vi "Export File - Tx XML.vi"(6 "RootNode":refnum<k24>, 7 "Tx Packets":T1 {"Tx Packet Data"."Endianness" items=["big-endian"=0, "little-endian"=2]}, 8 "error in (no error)":errorcluster, 11 "XmlDocument in":refnum<k24>) -> (0 "error out":errorcluster, 3 "XmlDocument out":refnum<k24>)   [LabVIEW 2016, in "UDP-Custom-Device System Explorer.lvlib"]
uses:
  UDP-Custom-Device System Explorer.lvlib
  System.Xml
  Types/XML - New/ImpExp - Tx Packets Data.ctl
  <vilib>/NI Veristand/Custom Device API/Custom Device Item Info.ctl
  Types/XML - New/ImpExp - Tx Packet Data.ctl
  Shared/Types/Shared - Channel Data Type.ctl
  Shared/Types/Shared - Buffered.PacketInfo.ctl
  Shared/Types/Shared - Pointer Encoding.ctl
  Types/XML - New/ImpExp - Packet Headers.ctl
  <vilib>/NI VeriStand/Custom Device API/Custom Device API.lvlib
  Shared/UDP-Custom-Device Shared.lvlib
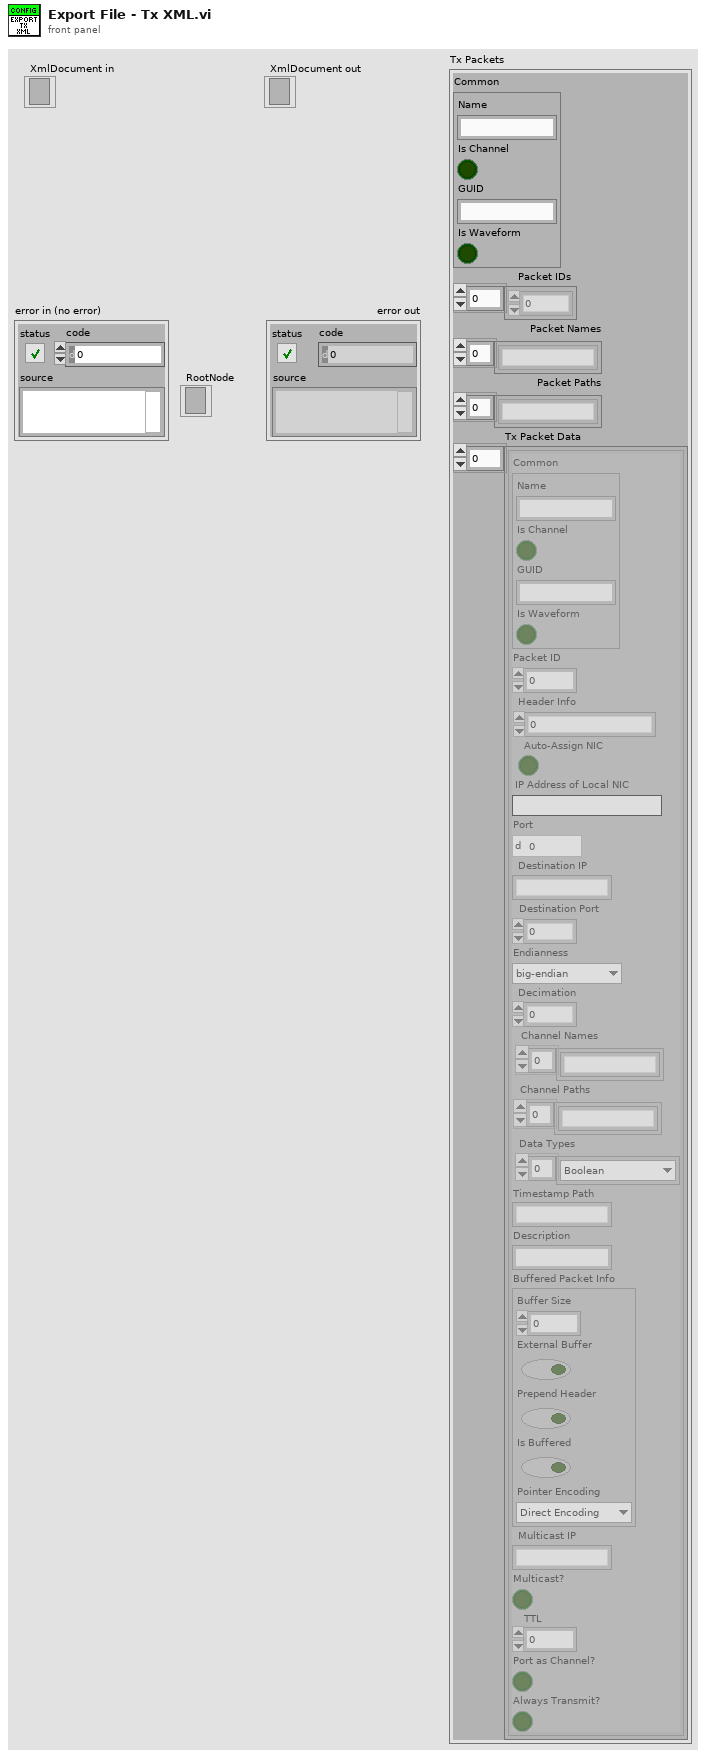
[diagram p1: front panel]
types:
  T1 = typedef "UDP-Custom-Device System Explorer.lvlib/ImpExp - Tx Packets Data.ctl" = cluster{"Common":T2, "Packet IDs":i32[], "Packet Names":string[], "Packet Paths":string[], "Tx Packet Data":T3[]}
  T2 = typedef "Custom Device API.lvlib/Custom Device Item Info.ctl" = cluster{"Name":string, "Is Channel":bool, "GUID":string, "Is Waveform":bool}
  T3 = typedef "UDP-Custom-Device System Explorer.lvlib/ImpExp - Tx Packet Data.ctl" = cluster{"Common":T2, "Packet ID":i32, "Header Info":u32, "Auto-Assign NIC":bool, "IP Address of Local NIC":string, "Port":u16, "Destination IP":string, "Destination Port":u16, "Endianness":u16, "Decimation":u16, "Channel Names":string[], "Channel Paths":string[], "Data Types":T4[], "Timestamp Path":string, "Description":string, "Buffered Packet Info":T5, "Multicast IP":string, "Multicast?":bool, "TTL":u16, "Port as Channel?":bool, "Always Transmit?":bool}
  T4 = typedef "UDP-Custom-Device Shared.lvlib/Shared - Channel Data Type.ctl" = enum16{"Boolean", "Single", "Double", "I8", "I16", "I32", "I64", "U8", "U16", "U32", "U64"}
  T5 = typedef "UDP-Custom-Device Shared.lvlib/Shared - Buffered.PacketInfo.ctl" = cluster{"Buffer Size":i32, "External Buffer":bool, "Prepend Header":bool, "Is Buffered":bool, "Pointer Encoding":T6}
  T6 = typedef "UDP-Custom-Device Shared.lvlib/Shared - Pointer Encoding.ctl" = enum16{"Direct Encoding", "Conversion Encoding"}
  T7 = typedef "UDP-Custom-Device System Explorer.lvlib/ImpExp - Packet Headers.ctl" = cluster{"Packet Name":string, "Packet ID":string, "Packet Path":string}
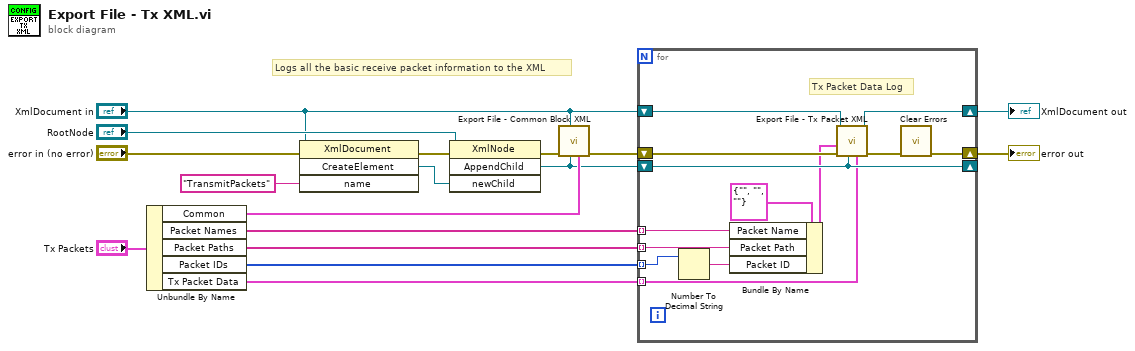
[diagram p0: block diagram]
diagram:
  # "Logs all the basic receive packet information to the XML"
  n1 = Unbundle By Name("Tx Packets") -> ("Common"=w10:T2, "Packet Names"=w6:string[], "Packet Paths"=w5:string[], "Packet IDs"=w4:i32[], "Tx Packet Data"=w3:T3[])
  n2 = invoke class="XmlDocument" method="CreateElement"(reference="XmlDocument in", error in="error in (no error)", "name"="TransmitPackets" ("Tag Name")) -> (error out=w15:errorcluster, "CreateElement"=w16:refnum<k24>)  [unwired: 1 in, 2 out]
  n3 = invoke class="XmlNode" method="AppendChild"(reference="RootNode", error in=w15, "newChild"=w16) -> (error out=w14:errorcluster, "AppendChild"=w7:refnum<k24>)  [unwired: 1 in, 2 out]
  n4 = call "Export File - Common Block XML.vi"("Common"=w10, "RootNode in"=w7, "XmlDocument in"="XmlDocument in", "error in (no error)"=w14) -> ("error out"=w8:errorcluster)  [unwired: 7 in]
  n5 = for {
    shift-right: [w18] -> w1
    shift-left: w8 -> [w25]
    shift-right: [w23] -> w2
    shift-left: "XmlDocument in" -> [w24]
    tunnel: w6 -> [w29] mode=indexing
    tunnel: w4 -> [w28] mode=indexing
    shift-right: [w22] -> _
    shift-left: w7 -> [w22]
    tunnel: w3 -> [w21] mode=indexing
    tunnel: w5 -> [w26] mode=indexing
    # "Tx Packet Data Log"
    n6 = Number To Decimal String(number=w28) -> (decimal integer string=w27:string)  [unwired: 1 in]
    n7 = Bundle By Name(cluster=T7 {"Packet Name"="", "Packet ID"="", "Packet Path"=""} ("Rx Packet XML Data"), "Packet Name"=w29, "Packet Path"=w26, "Packet ID"=w27) -> (w20:T7)
    n8 = call "Export File - Tx Packet XML.vi"("Tx Packet"=w21, "RootNode"=w22, "error in (no error)"=w25, "Tx Packet Header Data"=w20, "XmlDocument in"=w24) -> ("error out"=w19:errorcluster, "XmlDocument out"=w23:refnum<k24>)  [unwired: 5 in]
    n9 = call <vilib>:"Clear Errors.vi"("error in (no error)"=w19) -> ("error out"=w18:errorcluster)  [unwired: 5 in, 1 out]
  }
  "error out" <- w1
  "XmlDocument out" <- w2
